vi "FTW-Test-JSON-Units.vi"() -> (0 "Test Result":errorcluster)   [LabVIEW 2018]
uses:
  87a98d92-514c-4bc8-bca1-9e9f7e24a02c.vi
  3efb5aab-5bf0-4530-a08b-e186304dc382.vi
  source/JSON/core/FTW-JSON-Core-EncodingFlags.vi
  source/Reflection/FTW-Reflection-Type.vi
  source/JSON/FTW-JSON-Parse.vi
  source/container/FTW-Container-GetFlattenedValue.vi
  448beade-a94e-4925-9c2c-2f7e5f6d8622.vi
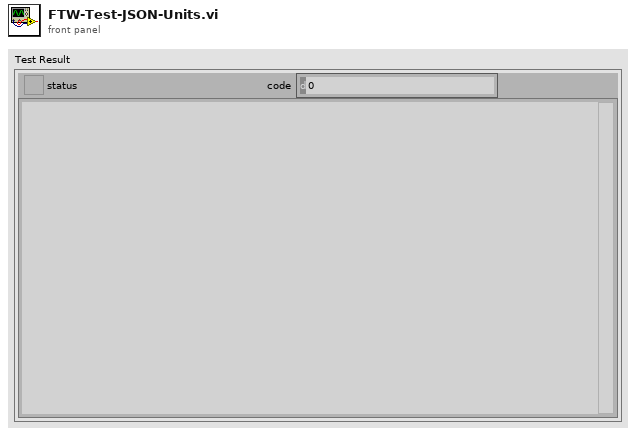
[diagram p1: front panel]
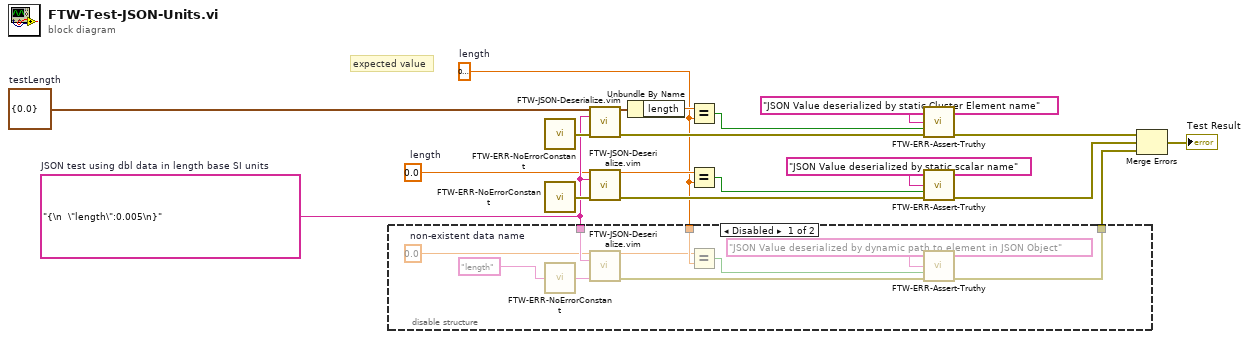
[diagram p0: block diagram]
diagram:
  w1 = dbl[unit] 0.005  # length
  w2 = dbl[unit] 0.0  # length
  w3 = cluster{"length":dbl[unit]} {"length"=0.0}  # testLength
  w14 = "{\n  \"length\":0.005\n}"  # JSON test using dbl data in length base SI units
  # "expected value"
  n1 = disable-structure shown="Disabled" {
    disable-tunnel: w14 -> [w28 _]
    disable-tunnel: [w26 _] -> w13
    disable-tunnel: w1 -> [w23 _]
    frame Disabled {
      w20 = dbl[unit] 0.0  # non-existent data name
      n2 = call "FTW-ERR-NoErrorConstant.vi"() -> ()  [unwired: 1 out]
      n3 = call "FTW-JSON-Deserialize.vim"("Type In"=w20, "JSON String"=w28, "error in"="length" ("Element Path")) -> ("Type Out"=w21:dbl[unit], "error out"=w27:errorcluster)  [unwired: 11 in]
      n4 = Equal?(x=w21, y=w23) -> (x = y?=w25:bool)
      n5 = call "FTW-ERR-Assert-Truthy.vi"("Assertion"="JSON Value deserialized by dynamic path to element in JSON Object", "Assertion holds true?"=w25, "error in"=w27) -> ("error out"=w26:errorcluster)  [unwired: 12 in]
    }
    frame Enabled {
    }
  }
  n6 = call "FTW-ERR-NoErrorConstant.vi"() -> ("no error"=w18:errorcluster)
  n7 = call "FTW-ERR-NoErrorConstant.vi"() -> ("no error"=w17:errorcluster)
  n8 = call "FTW-JSON-Deserialize.vim"("Type In"=w3, "JSON String"=w14, "error in"=w18) -> ("Type Out"=w19:cluster{"length":dbl[unit]}, "error out"=w8:errorcluster)  [unwired: 11 in]
  n9 = call "FTW-JSON-Deserialize.vim"("Type In"=w2, "JSON String"=w14, "error in"=w17) -> ("Type Out"=w15:dbl[unit], "error out"=w11:errorcluster)  [unwired: 11 in]
  n10 = Unbundle By Name(w19) -> ("length"=w16:dbl[unit])
  n11 = Equal?(x=w16, y=w1) -> (x = y?=w9:bool)
  n12 = Equal?(x=w15, y=w1) -> (x = y?=w12:bool)
  n13 = call "FTW-ERR-Assert-Truthy.vi"("Assertion"="JSON Value deserialized by static Cluster Element name", "Assertion holds true?"=w9, "error in"=w8) -> ("error out"=w7:errorcluster)  [unwired: 12 in]
  n14 = call "FTW-ERR-Assert-Truthy.vi"("Assertion"="JSON Value deserialized by static scalar name", "Assertion holds true?"=w12, "error in"=w11) -> ("error out"=w10:errorcluster)  [unwired: 12 in]
  n15 = Merge Errors(w7, w10, w13) -> (→"Test Result":errorcluster)
